vi "File.vi"(6 "Ini_State":T2, 8 "error in":errorcluster caption="entrée d'erreur", 11 "Valeur Write":T1) -> (0 "error out":errorcluster caption="sortie d'erreur", 3 "Valeur Read":T1)   [LabVIEW 2020]
doc: "Gestion du fichier XML INI"
uses:
  Ctrl/Ctrl_INI_state.ctl
  Ctrl/Ctrl_data_ini.ctl
  <vilib>/Utility/xml.llb/Read From XML File(string).vi
  <vilib>/Utility/xml.llb/Write to XML File(string).vi
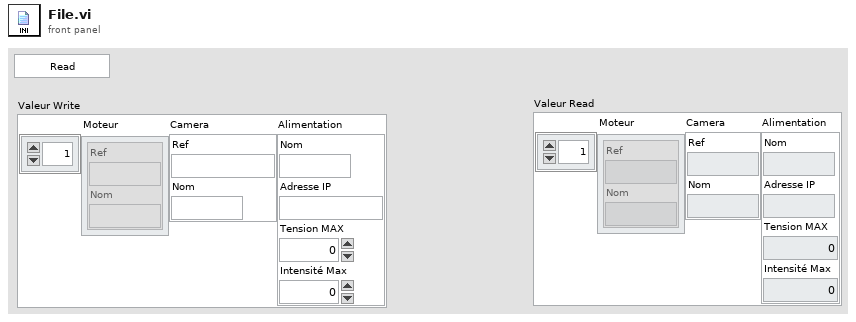
[diagram p1: front panel]
types:
  T1 = typedef "Ctrl_data_ini.ctl" = cluster{"Moteur":cluster{"Ref":string, "Nom":string}[], "Camera":cluster{"Ref":string, "Nom":string}, "Alimentation":cluster{"Nom ":string, "Adresse IP ":string, "Tension MAX":u8, "Intensité Max":dbl}}
  T2 = typedef "Ctrl_INI_state.ctl" = enum16{"Read", "Write"}
  T3 = enum16{"open", "replace", "create", "open or create", "replace or create", "replace or create with confirmation"}
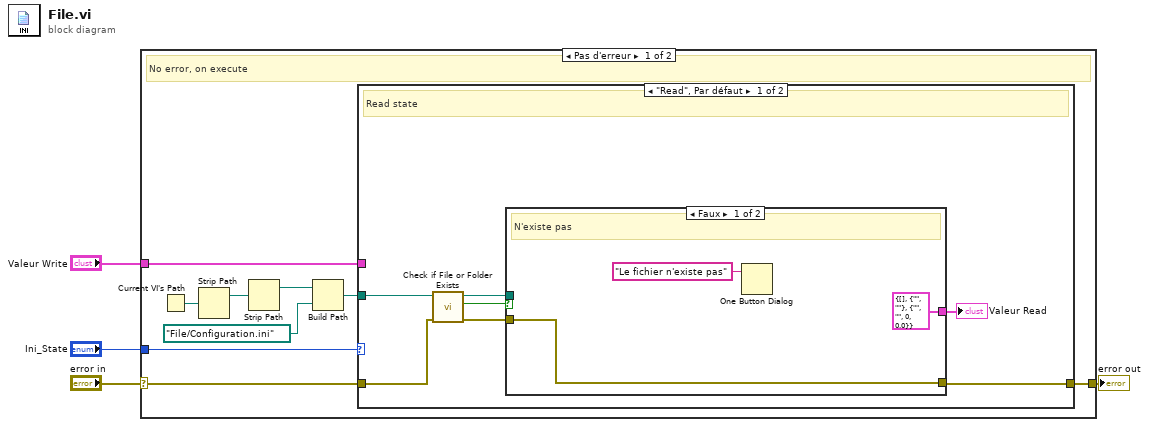
[diagram p0: block diagram]
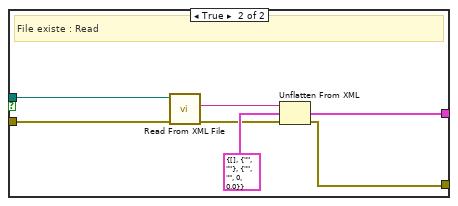
[diagram p2: hidden frame]
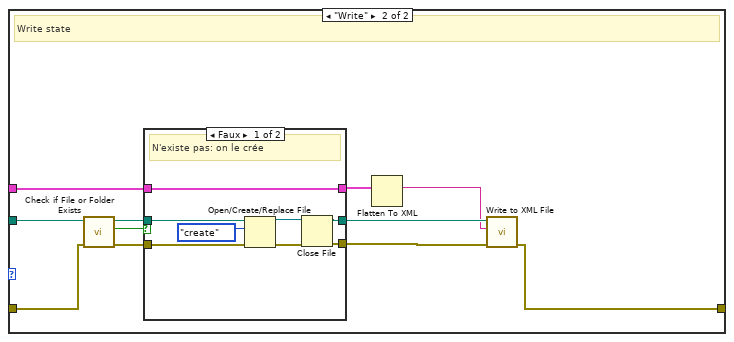
[diagram p3: hidden frame]
diagram:
  n1 = case shown="Pas d'erreur" "error in" {
    selector: "error in" -> [w13 w53]
    tunnel: [w12 w53] -> w3
    tunnel: "Ini_State" -> [w11 _]
    tunnel: "Valeur Write" -> [w5 _]
    frame No Error {
      # "No error, on execute"
      n2 = Current VI's Path() -> (path=w10:path)
      n3 = Strip Path(path=w10) -> (stripped path=w9:path)  [unwired: 1 out]
      n4 = Strip Path(path=w9) -> (stripped path=w8:path)  [unwired: 1 out]
      n5 = Build Path(base path=w8, name or relative path=path "File/Configuration.ini" ("nom ou chemin relatif")) -> (appended path=w6:path)
      n6 = case shown="\"Read\", Par défaut" w11 {
        tunnel: w13 -> [w19 w41]
        tunnel: [w20 w32] -> w12
        tunnel: w6 -> [w15 w37]
        tunnel: w5 -> [_ w36]
        frame "Read", Default {
          # "Read state"
          n7 = call <vilib>:"Check if File or Folder Exists.vi"("error in (no error)"=w19, "path"=w15) -> ("error out"=w17:errorcluster, "file or folder exists?"=w16:bool, "dup path"=w18:path)  [unwired: 7 in]
          n8 = case shown="Faux" w16 {
            tunnel: [w23 w27] -> w20
            tunnel: w18 -> [_ w26]
            tunnel: w17 -> [w23 w25]
            tunnel: [T1 {"Moteur"=[], "Camera"={"Ref"="", "Nom"=""}, "Alimentation"={"Nom "="", "Adresse IP "="", "Tension MAX"=0, "Intensité Max"=0.0}} ("Database") w24] -> w14
            frame False {
              # "N'existe pas"
              n9 = One Button Dialog(message="Le fichier n'existe pas") -> ()  [unwired: 1 in, 1 out]
            }
            frame True {
              # "File existe : Read"
              n10 = call-poly <vilib>:"Read From XML File.vi"("error in (no error)"=w25, "XML File Path"=w26) -> ("error out"=w28:errorcluster, "XML Elements"=w30:string)  [unwired: 7 in, 1 out]
              n11 = Unflatten From XML(xml string=w30, type=T1 {"Moteur"=[], "Camera"={"Ref"="", "Nom"=""}, "Alimentation"={"Nom "="", "Adresse IP "="", "Tension MAX"=0, "Intensité Max"=0.0}} ("Database"), error in (no error)=w28) -> (value=w24:T1, error out=w27:errorcluster)
            }
          }
          "Valeur Read" <- w14
        }
        frame "Write" {
          # "Write state"
          n12 = call <vilib>:"Check if File or Folder Exists.vi"("error in (no error)"=w41, "path"=w37) -> ("error out"=w39:errorcluster, "file or folder exists?"=w38:bool, "dup path"=w40:path)  [unwired: 7 in]
          n13 = case shown="Faux" w38 {
            tunnel: w40 -> [w43 w50]
            tunnel: w39 -> [w48 w51]
            tunnel: w36 -> [w45 w52]
            tunnel: [w45 w52] -> w35
            tunnel: [w44 w51] -> w33
            tunnel: [w42 w50] -> w34
            frame False {
              # "N'existe pas: on le crée"
              n14 = Open/Create/Replace File(file path (use dialog)=w43, error in=w48, operation (0:open)=T3."create" ("opération (0 : open)")) -> (refnum out=w46:refnum<file>, error out=w47:errorcluster)  [unwired: 3 in, 1 out]
              n15 = Close File(refnum=w46, error in=w47) -> (path=w42:path, error out=w44:errorcluster)
            }
            frame True {
              # "File existe : on ne fait rien"
            }
          }
          n16 = Flatten To XML(6:w35) -> (2:w31:string)
          n17 = call-poly <vilib>:"Write to XML File.vi"("error in (no error)"=w33, "XML Input"=w31, "XML File Path"=w34) -> ("error out"=w32:errorcluster)  [unwired: 6 in, 2 out]
        }
      }
    }
    frame Error {
      # "Error on laisse passer le flux"
    }
  }
  "error out" <- w3
